vi "HFRR ADV v06.vi"() -> ()   [LabVIEW 2025] (continued)
        n2251 = case shown="\"Acquire\"" w2733 {
          tunnel: w2735 -> [_ w2966]
          frame Default {
            w2965 = 0.0 ("output")
            n2252 = local write "PID-out"(w2965) -> ()
            n2253 = local write "Frequency ( Hz )"(w2965) -> ()
          }
          frame "Acquire" {
            n2254 = stacked-sequence {
              frame #0 {
                n2255 = local read "clk"() -> (w2986:dbl)
                n2256 = local read "Save"() -> (w2982:bool)
                n2257 = Equal?(x=w2986, y=0.0) -> (x = y?=w2983:bool)
                n2258 = case shown="False" "RUN" {
                  tunnel: [w2991 w2999] -> w2969
                  frame False {
                    w2991 = 0.0
                    n2259 = local write "Reinit PID"(TRUE) -> ()
                    n2260 = property on="Stroke" class="DigNum (strict)"("Visible"=TRUE) -> ()  [unwired: 2 in, 2 out]
                    n2261 = property on="Stroke 2" class="DigNum (strict)"("Visible"=FALSE) -> ()  [unwired: 2 in, 2 out]
                    n2262 = local write "String 14"("Test will autostart once parameters reach the set value." ("String 14")) -> ()
                    n2263 = local write "Old Pid Val"(w2991) -> ()
                  }
                  frame True {
                    n2264 = property on="Stroke 2" class="DigNum (strict)"("Visible"=TRUE) -> ()  [unwired: 2 in, 2 out]
                    n2265 = property on="Stroke" class="DigNum (strict)"("Visible"=FALSE) -> ()  [unwired: 2 in, 2 out]
                    n2266 = property on="STOP 2" class="Bool (strict)"("Disabled"=u8 2) -> ()  [unwired: 2 in, 2 out]
                    n2267 = property on="RUN" class="Bool (strict)"("Visible"=TRUE) -> ()  [unwired: 2 in, 2 out]
                    n2268 = local read "PID Ref"() -> (w3010:bool)
                    n2269 = case shown="True" w3010 {
                      tunnel: [w3011 w3027] -> w3009
                      frame False {
                        n2270 = local read "Old Pid Val"() -> (w3011:dbl)
                      }
                      frame True {
                        n2271 = local read "Set Hz"() -> (w3020:dbl)
                        n2272 = local read "Frequency"() -> (w3031:dbl)
                        n2273 = Add(x=w3020, y=10.0) -> (x+y=w3029:dbl)
                        n2274 = Add(x=w3020, y=-10.0 ("Offset")) -> (x+y=w3038:dbl)
                        n2275 = Add(x=w3020, y=-10.0) -> (x+y=w3030:dbl)
                        n2276 = In Range and Coerce(upper limit=w3029, x=w3031, lower limit=w3030) -> (coerced(x)=w3019:dbl)  [unwired: 1 out]
                        n2277 = Or(x="Reinit PID", y="Reinit PID") -> (x .or. y?=w3028:bool)
                        n2278 = Multiply(x=w3038, y=0.1 ("Gain")) -> (x*y=w3017:dbl)
                        n2279 = local read "Elapsed time"() -> (w3024:dbl)
                        n2280 = local read "SPEED OUT:"() -> (w3039:dbl)
                        n2281 = Add(x=w3017, y=1.5) -> (x+y=w3015:dbl)
                        n2282 = call-poly <vilib>:"PID.vi"("reinitialize? (F)"=w3028, "output range"=cluster{"output high":dbl, "output low":dbl} {"output high"=1.0, "output low"=-1.0}, "PID gains"=T10 {"proportional gain (Kc)"=0.0005, "integral time (Ti, min)"=0.001, "derivative time (Td, min)"=0.0} ("Motor PID"), "process variable"=w3019, "setpoint"=w3020) -> ("output"=w3018:dbl)  [unwired: 5 in, 1 out]
                        n2283 = Multiply(x=w3015, y=w3039) -> (x*y=w3014:dbl)
                        n2284 = Greater?(x=w3024, y=0.05) -> (0:w3023:bool)
                        n2285 = case shown="True" w3023 {
                          tunnel: w3018 -> [_ w3041]
                          tunnel: [0.0 ("output") w3041] -> w3021
                          frame False {
                          }
                          frame True {
                            n2286 = local write "Reinit PID"(FALSE ("Reinit PID")) -> ()
                          }
                        }
                        n2287 = Multiply(x=w3014, y=0.8) -> (x*y=w3013:dbl)
                        n2288 = Add(x=w3013, y=w3021) -> (x+y=w3026:dbl)
                        n2289 = flat-sequence {
                          tunnel: [w3044] -> w3027
                          tunnel: w3026 -> [w3044]
                          frame #0 {
                            n2290 = local write "PID Ref"(FALSE ("PID Ref")) -> ()
                          }
                        }
                      }
                    }
                    "Old Pid Val" <- w3009
                    n2291 = local write "String 14"(" Running....." ("String 14")) -> ()
                    n2292 = local read "Set Hz"() -> (w3006:dbl)
                    n2293 = call <vilib>:"Uniform White Noise Waveform.vi"() -> ("signal out"=w3005:waveform(dbl))  [unwired: 10 in, 1 out]
                    n2294 = local read "Freq"() -> (w2998:dbl)
                    n2295 = Add(x=w3006, y=w3005) -> (x+y=w3004:waveform(dbl))
                    n2296 = Multiply(x=w3004, y=ext 0.1) -> (x*y=w3000:waveform(ext))
                    n2297 = Multiply(x=w2998, y=0.9) -> (x*y=w3001:dbl)
                    n2298 = Add(x=w3000, y=w3001) -> (x+y=w2999:waveform(ext))
                  }
                }
                n2299 = And(x=w2983, y=w2982) -> (x .and. y?=w2984:bool)
                n2300 = Not(x="Engage") -> (.not. x?=w2973:bool)
                n2301 = case shown="True" w2984 {
                  frame False {
                  }
                  frame True {
                    n2302 = local write "clk"(10.0 ("clk")) -> ()
                    n2303 = Get Date/Time In Seconds() -> (seconds since 1Jan1904=w3047:timestamp)
                    n2304 = To Double Precision Float(number=w3047) -> (double precision float=w3045:dbl)
                    n2305 = local write "acq timer"(w3045) -> ()
                    n2306 = local write "act save time"(w3045) -> ()
                  }
                }
                n2307 = call "Elapsed Time"("Time Target (s)"="Countdown", "Reset"=w2973) -> ("Elapsed Time (s)"=w2978:dbl, "Time has Elapsed"=w2976:bool)  [unwired: 10 in, 6 out]
                "Countdown 2" <- w2978
                n2308 = Subtract(x=w2978, y=2.0) -> (x-y=w2981:dbl)
                n2309 = Less?(x=w2981, y="Countdown") -> (x < y?=w2979:bool)
                n2310 = And(x=w2979, y=w2976) -> (x .and. y?=w2975:bool)
                n2311 = case shown="True" w2975 {
                  frame False {
                  }
                  frame True {
                    (unwired) dbl[] [] ("History Data")
                    n2312 = local write "Engage"(FALSE ("Engage")) -> ()
                    n2313 = local write "RUN"(TRUE ("RUN")) -> ()
                    n2314 = local read "Humidity ( %RH )"() -> (→"Rh Before":dbl)
                  }
                }
                n2315 = local read "Test \nStatus"() -> (w2971:bool)
                n2316 = Select(t=w2969, s=w2971, f=0.0) -> (s? t:f=w2970:dbl)
                n2317 = local write "Frequency ( Hz )"(w2970) -> ()
                n2318 = local write "Freq"(w2970) -> ()
              }
              frame #1 {
                w3070 = 1000000.0 ("x")
                # "Elapsed time\ncof\nstroke\nAir temp\nTemp\nHumidity"
                # "acq timer\n\nact save time"
                # "convert to microseconds"
                n2319 = local read "COUNT"() -> (w3053:i32)
                n2320 = local read "Rate"() -> (w3066:dbl)
                n2321 = Divide(x=w3070, y=w3066) -> (x/y=w3071:dbl)
                n2322 = Greater Or Equal?(x=w3053, y=250) -> (x >= y?=w3052:bool)
                n2323 = Get Date/Time In Seconds() -> (seconds since 1Jan1904=w3073:timestamp)
                n2324 = case shown="True" w3052 {
                  frame False {
                    n2325 = local read "COUNT"() -> (w3074:i32)
                    n2326 = Increment(x=w3074) -> (x+1=w3075:i32)
                    n2327 = local write "COUNT"(w3075) -> ()
                  }
                  frame True {
                    n2328 = local write "COUNT"(0 ("COUNT")) -> ()
                  }
                }
                n2329 = local read "Samplingtime 2"() -> (w3051:dbl)
                n2330 = local read "act save time"() -> (w3068:dbl)
                n2331 = Divide(x=w3071, y=w3070) -> (x/y=w3069:dbl)
                n2332 = To Double Precision Float(number=w3073) -> (double precision float=w3062:dbl)
                n2333 = Add(x=w3068, y=w3051) -> (x+y=w3067:dbl)
                n2334 = local read "acq timer"() -> (w3072:dbl)
                n2335 = local read "COUNT"() -> (w3055:i32)
                n2336 = Greater Or Equal?(x=w3062, y=w3067) -> (x >= y?=w3050:bool)
                n2337 = Multiply(x=w3069, y=w3055) -> (x*y=w3061:dbl)
                n2338 = Subtract(x=w3062, y=w3072) -> (x-y=w3064:dbl)
                n2339 = local read "Save"() -> (w3065:bool)
                n2340 = Add(x=w3064, y=w3061) -> (x+y=w3048:dbl)
                "Elapsed time 3" <- w3048
                n2341 = And(x=w3050, y=w3065) -> (x .and. y?=w3063:bool)
                n2342 = Divide(x=w3048, y=60.0) -> (x/y=w3059:dbl)
                n2343 = local read "Test \nStatus"() -> (w3049:bool)
                n2344 = local read "clk"() -> (w3056:dbl)
                n2345 = case shown="True" w3063 {
                  tunnel: w3062 -> [_ w3164]
                  tunnel: [FALSE ("Boolean 2") TRUE ("Boolean 2")] -> _
                  frame False {
                  }
                  frame True {
                    w3111 = ";" ("Substring")
                    # "Pid out/\nFreq response value"
                    n2346 = local read "FILE"() -> (w3105:string)
                    n2347 = call "file check.vi"("file name in"=w3105) -> ("error out"=w3108:errorcluster, "file name out"=w3103:string)  [unwired: 9 in]
                    n2348 = call "FILE PATH CREATION.vi"("error in"=w3108, "FILE NAME :"=w3103) -> ("FILE OUT"=w3106:path)  [unwired: 8 in, 1 out]
                    n2349 = Concatenate Strings(w3103, ".dgf" ("Substring")) -> (w3107:string)
                    n2350 = local write "act save time"(w3164) -> ()
                    n2351 = local read "Set Strk"() -> (w3135:dbl)
                    n2352 = local read "Stroke"() -> (w3126:dbl)
                    n2353 = local read "FF 2"() -> (w3122:dbl)
                    "Frictional Force ( N )" <- w3122
                    "Frictional Force ( N )" <- w3122
                    n2354 = Build Path(base path=w3106, name or relative path=w3107) -> (appended path=w3102:path)
                    n2355 = local write "FF 3"(w3122) -> ()
                    n2356 = Subtract(x=w3126, y=w3135) -> (x-y=w3132:dbl)
                    n2357 = local read "COF 2"() -> (w3117:dbl)
                    "cof" <- w3117
                    "Coefficient of Friction" <- w3117
                    "COF 4" <- w3117
                    "Coefficient of Friction" <- w3117
                    n2358 = local write "COF 3"(w3117) -> ()
                    n2359 = Multiply(x=w3132, y=0.05) -> (x*y=w3134:dbl)
                    n2360 = local read "TEMP"() -> (w3121:dbl)
                    "Temp" <- w3121
                    "Temperature ( Deg C )" <- w3121
                    n2361 = Add(x=w3134, y=w3135) -> (x+y=w3115:dbl)
                    "Stroke Ln" <- w3115
                    "Disp" <- w3115
                    n2362 = local read "ecr"() -> (w3118:dbl)
                    "ecr 2" <- w3118
                    "Electrical Contact Resistance ( % )" <- w3118
                    "ecr 4" <- w3118
                    n2363 = local read "Humidity ( %RH )"() -> (w3120:dbl)
                    "Humidity ( %RH )" <- w3120
                    "Humidity ( %RH )" <- w3120
                    n2364 = local read "Frequency ( Hz )"() -> (w3128:dbl)
                    n2365 = local read "Elapsed time"() -> (w3157:dbl)
                    n2366 = local read "AIR TEMP"() -> (w3125:dbl)
                    n2367 = local write "ecr 3"(w3118) -> ()
                    n2368 = local read "PID-out"() -> (w3131:dbl)
                    n2369 = local write "Temperature ( Deg C )"(w3121) -> ()
                    n2370 = local write "Electrical Contact Resistance ( % )"(w3118) -> ()
                    n2371 = Number To Fractional String(number=w3115, width (-)=i16 9 ("precision (6)"), precision (6)=i16 6) -> (F-format string=w3150:string)  [unwired: 1 in]
                    n2372 = Number To Fractional String(number=w3125, width (-)=i16 9 ("precision (6)"), precision (6)=i16 3) -> (F-format string=w3149:string)  [unwired: 1 in]
                    n2373 = Number To Fractional String(number=w3121, width (-)=i16 9 ("precision (6)"), precision (6)=i16 3) -> (F-format string=w3146:string)  [unwired: 1 in]
                    n2374 = Number To Fractional String(number=w3120, width (-)=i16 9 ("precision (6)"), precision (6)=i16 3) -> (F-format string=w3143:string)  [unwired: 1 in]
                    n2375 = Number To Fractional String(number=w3118, width (-)=i16 9 ("precision (6)"), precision (6)=i16 3) -> (F-format string=w3140:string)  [unwired: 1 in]
                    n2376 = Number To Fractional String(number=w3131, width (-)=i16 9 ("precision (6)"), precision (6)=i16 3) -> (F-format string=w3136:string)  [unwired: 1 in]
                    n2377 = Number To Fractional String(number=w3128, width (-)=i16 9 ("precision (6)"), precision (6)=i16 3) -> (F-format string=w3127:string)  [unwired: 1 in]
                    n2378 = Number To Fractional String(number=w3117, width (-)=i16 9 ("precision (6)"), precision (6)=i16 6) -> (F-format string=w3158:string)  [unwired: 1 in]
                    n2379 = Number To Fractional String(number=w3157, width (-)=i16 14 ("precision (6)"), precision (6)=i16 3) -> (F-format string=w3159:string)  [unwired: 1 in]
                    n2380 = Bundle("y"=1.02, w3115, "y"=0.98) -> (w3119:cluster{"y":dbl, dbl, "y":dbl})  [unwired: 1 in]
                    n2381 = Number To Fractional String(number="Ambient Humidity :", width (-)=i16 9 ("precision (6)"), precision (6)=i16 6) -> (F-format string=w3109:string)  [unwired: 1 in]
                    n2382 = local read "RUN"() -> (w3116:bool)
                    n2383 = case shown="True" w3116 {
                      tunnel: w3119 -> [_ w3169]
                      tunnel: w3115 -> [_ w3168]
                      tunnel: w3115 -> [_ w3167]
                      tunnel: w3115 -> [_ w3166]
                      frame False {
                      }
                      frame True {
                        "Stroke ( mm )" <- w3169
                        "Stroke ( mm )" <- w3169
                        "Stroke 4" <- w3168
                        "Stroke 3" <- w3167
                        "Stroke 2" <- w3166
                      }
                    }
                    n2384 = Concatenate Strings(w3159, w3111, w3158, w3111, w3150, w3111, w3149, w3111, w3146, w3111, w3143, w3111, w3140, w3111, w3136, w3111, w3127, w3111, w3109, "\r") -> (w3156:string)
                    n2385 = call <vilib>:"Write Characters To File.vi"("append to file? (new file:F)"=TRUE, "character string"=w3156, "file path (dialog if empty)"=w3102) -> ()  [unwired: 2 in, 1 out]
                    "refresh flag" <- TRUE ("refresh flag")
                  }
                }
                n2386 = Equal?(x=w3056, y=10.0) -> (x = y?=w3058:bool)
                n2387 = case shown="True" w3049 {
                  tunnel: w3059 -> [_ w3082]
                  tunnel: w3064 -> [_ w3093]
                  tunnel: [0.0 w3089] -> _
                  tunnel: w3058 -> [_ w3088]
                  tunnel: [0.0 w3087] -> _
                  tunnel: w3048 -> [_ w3087]
                  tunnel: w3062 -> [w3078 _]
                  frame False {
                    n2388 = local write "acq timer"(w3078) -> ()
                    n2389 = local write "Test Duration Status"(0.0 ("Test Duration Status")) -> ()
                  }
                  frame True {
                    n2390 = local read "Set Hz"() -> (w3090:dbl)
                    n2391 = local write "Elapsed time"(w3082) -> ()
                    n2392 = local read "test time"() -> (w3081:dbl)
                    n2393 = Multiply(x=w3093, y=w3090) -> (x*y=w3092:dbl)
                    n2394 = case shown="False" w3088 {
                      tunnel: w3092 -> [w3094 _]
                      tunnel: [w3094 1.0] -> w3089
                      frame False {
                        n2395 = local write "Cycles elapsed"(w3094) -> ()
                      }
                      frame True {
                      }
                    }
                    n2396 = Greater?(x=w3082, y=w3081) -> (0:w3091:bool)
                    n2397 = Subtract(x=w3081, y=w3082) -> (x-y=w3086:dbl)
                    "time" <- w3086
                    n2398 = case shown="True" w3091 {
                      frame False {
                      }
                      frame True {
                        n2399 = local write "RUN"(FALSE ("OK Button 2")) -> ()
                        n2400 = property on="STOP 2" class="Bool (strict)"("Disabled"=u8 0) -> ()  [unwired: 2 in, 2 out]
                        n2401 = local read "Humidity ( %RH )"() -> (→"Rh After":dbl)
                        n2402 = local write "Heater Button"(FALSE ("Heater Button")) -> ()
                        n2403 = local write "Humidity"(FALSE ("Humidity")) -> ()
                      }
                    }
                    n2404 = local write "Time Remaining"(w3086) -> ()
                    n2405 = Divide(x=w3082, y=w3081) -> (x/y=w3085:dbl)
                    n2406 = Multiply(x=w3085, y=100.0) -> (x*y=w3083:dbl)
                    n2407 = local write "Test Duration Status"(w3083) -> ()
                  }
                }
              }
              frame #2 {
                n2408 = case shown="True" "Heater Button" {
                  tunnel: [0.0 ("output") w3191] -> w3170
                  frame False {
                    w3172 = TRUE ("tmpchk")
                    n2409 = local read "TEMP"() -> (w3173:dbl)
                    n2410 = local write "Temp ini"(w3173) -> ()
                    n2411 = local write "Reset 4"(w3172) -> ()
                    n2412 = local write "tmpchk"(w3172) -> ()
                    n2413 = local write "reinit"(TRUE ("reinit")) -> ()
                  }
                  frame True {
                    # "Logic to turn off\nthe heater when \ntemp is not rising.\nTime - 60 sec\nDelta t- 5°c"
                    n2414 = local read "Temp ini"() -> (w3179:dbl)
                    n2415 = Less?(x=w3179, y=53.0) -> (x < y?=w3177:bool)
                    n2416 = And(x="tmpchk", y=w3177) -> (x .and. y?=w3180:bool)
                    n2417 = case shown="True" w3180 {
                      frame False {
                      }
                      frame True {
                        n2418 = call "Elapsed Time8"("Time Target (s)"=300.0, "Reset"="Reset 4") -> ("Time has Elapsed"=w3196:bool)  [unwired: 10 in, 7 out]
                        n2419 = flat-sequence {
                          tunnel: w3196 -> [_]
                          frame #0 {
                            n2420 = local write "Reset 4"(FALSE ("Reset 4")) -> ()
                          }
                        }
                        n2421 = case shown="True" w3196 {
                          frame False {
                          }
                          frame True {
                            n2422 = local read "Temp ini"() -> (w3203:dbl)
                            n2423 = Add(x=w3203, y=5.0) -> (x+y=w3201:dbl)
                            n2424 = local read "TEMP"() -> (w3204:dbl)
                            n2425 = Greater?(x=w3204, y=w3201) -> (0:w3202:bool)
                            n2426 = case shown="False" w3202 {
                              frame False {
                                n2427 = local write "Heater Button"(FALSE ("Heater Button")) -> ()
                              }
                              frame True {
                                n2428 = local write "tmpchk"(FALSE ("tmpchk")) -> ()
                              }
                            }
                          }
                        }
                      }
                    }
                    n2429 = local read "Set Temp"() -> (w3188:dbl)
                    n2430 = local read "TEMP"() -> (w3182:dbl)
                    n2431 = call-poly <vilib>:"PID.vi"("reinitialize? (F)"="reinit", "output range"="output range", "dt (s)"=-1.0, "PID gains"="Temp PID gains", "process variable"=w3182, "setpoint"=w3188) -> ("output"=w3185:dbl)  [unwired: 4 in, 1 out]
                    n2432 = Subtract(x=w3188, y=w3182) -> (x-y=w3190:dbl)
                    n2433 = Add(x=w3188, y=0.5) -> (x+y=w3186:dbl)
                    n2434 = Greater Or Equal?(x=w3182, y=w3186) -> ()  [unwired: 1 out]
                    n2435 = Select(t=0.0, s=FALSE, f=w3185) -> (s? t:f=w3184:dbl)
                    "PID output" <- w3184
                    n2436 = flat-sequence {
                      tunnel: w3184 -> [w3207]
                      tunnel: [w3207] -> w3191
                      frame #0 {
                        n2437 = local write "reinit"(FALSE ("reinit")) -> ()
                      }
                    }
                    n2438 = Bundle(w3190, "output"=w3184, "TEMP"=w3182) -> (→"gTEMP 3":cluster{dbl, "output":dbl, "TEMP":dbl})  [unwired: 1 in]
                  }
                }
                "PID-out" <- w3170
              }
              frame #3 {
                n2439 = local read "TEMP"() -> (w3209:dbl)
                n2440 = Greater Or Equal?(x=w3209, y="Set Temp 2") -> (x >= y?=w3214:bool)
                n2441 = case shown="True" w3214 {
                  tunnel: [FALSE TRUE] -> w3212
                  frame False {
                  }
                  frame True {
                  }
                }
                "Status 13" <- w3212
                n2442 = And(x=w3212, y="trip1 8") -> (x .and. y?=w3211:bool)
                n2443 = case shown="True" w3211 {
                  frame False {
                  }
                  frame True {
                    w3215 = FALSE ("OK Button 2")
                    n2444 = local write "RUN"(w3215) -> ()
                    n2445 = local write "Heater Button"(w3215) -> ()
                  }
                }
              }
            }
            n2446 = case shown="False" w2966 {
              frame False {
                n2447 = disable-structure shown="Enabled" {
                  frame Enabled {
                    n2448 = stacked-sequence {
                      frame #0 {
                        n2449 = local write "RUN"(FALSE ("OK Button 2")) -> ()
                      }
                      frame #1 {
                      }
                    }
                  }
                  frame Disabled {
                  }
                }
              }
              frame True {
              }
            }
          }
        }
        n2450 = local read "airtempflg"() -> (w2758:bool)
        n2451 = Or(x=w2758, y=w2756) -> (x .or. y?=w2759:bool)
        n2452 = Insert Into Array(array=string[] ["Air Temperature has reached set value,", "Humidity has reached set value,", "Sample Temperaturehas reached set value,", ""], index=0, new element="") -> (w2744:string[])
        n2453 = disable-structure shown="Disabled" {
          disable-tunnel: w2759 -> [w2836 _]
          disable-tunnel: w2754 -> [w2835 _]
          disable-tunnel: w2752 -> [w2834 _]
          frame Disabled {
            n2454 = Compound Arithmetic op=AND(w2836, w2835, w2834) -> ()  [unwired: 1 out]
            n2455 = case shown="True" {
              selector: _ -> [_ _]
              frame False {
              }
              frame True {
                w2837 = FALSE ("autostrtflg")
                n2456 = local write "RUN"(TRUE ("RUN")) -> ()
                n2457 = local write "autostrtflg"(w2837) -> ()
                n2458 = local write "autostart"(w2837) -> ()
                n2459 = local write "String 14"(" Running....." ("String 14")) -> ()
              }
            }
          }
          frame Enabled {
          }
        }
        n2460 = Build Array(w2749, w2748, w2747) -> (w2745:i32[])
        n2461 = for {
          tunnel: w2745 -> [w2887] mode=indexing
          tunnel: w2744 -> [w2886]
          shift-right: [w2883] -> w2743
          shift-left: "" -> [w2885]
          n2462 = Index Array(array=w2886, index=w2887) -> (element=w2884:string)
          n2463 = Concatenate Strings(w2884, w2885) -> (w2883:string)
        }
        n2464 = local write "autostart 2"(w2743) -> ()
        n2465 = local read "Reset Graph"() -> (w2732:bool)
        n2466 = case shown="True" w2732 {
          selector: w2732 -> [_ w2786]
          frame False {
          }
          frame True {
            w2800 = 0.0 ("X Scale.Range:Maximum")
            n2467 = Not(x=w2786) -> (.not. x?=w2785:bool)
            n2468 = local write "Reset Graph"(w2785) -> ()
            n2469 = property on="Electrical Contact Resistance ( % )" class="WFChart (strict)"("XScale.Maximum"=600.0 ("X Scale.Range:Maximum"), "XScale.Minimum"=0.0 ("X Scale.Range:Minimum"), "YScale.Maximum"=100.0 ("Y Scale.Range:Maximum"), "YScale.Minimum"=0.0 ("Y Scale.Range:Minimum")) -> ()  [unwired: 2 in, 2 out]
            n2470 = property on="Frictional Force ( N )" class="WFChart (strict)"("XScale.Maximum"=600.0 ("X Scale.Range:Maximum"), "XScale.Minimum"=0.0 ("X Scale.Range:Minimum"), "YScale.Maximum"=100.0 ("Y Scale.Range:Maximum"), "YScale.Minimum"=0.0 ("Y Scale.Range:Minimum")) -> ()  [unwired: 2 in, 2 out]
            n2471 = property on="Temperature ( Deg C )" class="WFChart (strict)"("XScale.Maximum"=600.0 ("X Scale.Range:Maximum"), "XScale.Minimum"=0.0 ("X Scale.Range:Minimum"), "YScale.Maximum"=100.0 ("Y Scale.Range:Maximum"), "YScale.Minimum"=0.0 ("Y Scale.Range:Minimum")) -> ()  [unwired: 2 in, 2 out]
            n2472 = property on="Humidity ( %RH )" class="WFChart (strict)"("XScale.Maximum"=600.0 ("X Scale.Range:Maximum"), "XScale.Minimum"=0.0 ("X Scale.Range:Minimum"), "YScale.Maximum"=100.0 ("Y Scale.Range:Maximum"), "YScale.Minimum"=0.0 ("Y Scale.Range:Minimum")) -> ()  [unwired: 2 in, 2 out]
            n2473 = property on="Stroke ( mm )" class="WFChart (strict)"("XScale.Maximum"=600.0 ("X Scale.Range:Maximum"), "XScale.Minimum"=0.0 ("X Scale.Range:Minimum"), "YScale.Maximum"=100.0 ("Y Scale.Range:Maximum"), "YScale.Minimum"=0.0 ("Y Scale.Range:Minimum")) -> ()  [unwired: 2 in, 2 out]
            n2474 = property on="Coefficient of Friction" class="WFChart (strict)"("XScale.Maximum"=600.0 ("X Scale.Range:Maximum"), "XScale.Minimum"=0.0 ("X Scale.Range:Minimum"), "YScale.Maximum"=100.0 ("Y Scale.Range:Maximum"), "YScale.Minimum"=0.0 ("Y Scale.Range:Minimum")) -> ()  [unwired: 2 in, 2 out]
            n2475 = property on="Electrical Contact Resistance ( % )" class="WFChart (strict)"("XScale.Minimum"=0.0 ("X Scale.Range:Minimum"), "XScale.Maximum"=600.0 ("X Scale.Range:Maximum"), "YScale.Minimum"=0.0 ("Y Scale.Range:Minimum"), "YScale.Maximum"=100.0 ("Y Scale.Range:Maximum")) -> ()  [unwired: 2 in, 2 out]
            n2476 = property on="Temperature ( Deg C )" class="WFChart (strict)"("XScale.Minimum"=0.0 ("X Scale.Range:Minimum"), "XScale.Maximum"=600.0 ("X Scale.Range:Maximum"), "YScale.Minimum"=0.0 ("Y Scale.Range:Minimum"), "YScale.Maximum"=100.0 ("Y Scale.Range:Maximum")) -> ()  [unwired: 2 in, 2 out]
            n2477 = property on="Coefficient of Friction" class="WFChart (strict)"("XScale.Minimum"=0.0 ("X Scale.Range:Minimum"), "XScale.Maximum"=600.0 ("X Scale.Range:Maximum"), "YScale.Maximum"=1.0 ("X Scale.Range:Minimum"), "YScale.Minimum"=0.0 ("X Scale.Range:Minimum")) -> ()  [unwired: 2 in, 2 out]
            n2478 = property on="Frictional Force ( N )" class="WFChart (strict)"("XScale.Maximum"=600.0 ("X Scale.Range:Maximum"), "XScale.Minimum"=w2800, "YScale.Maximum"=10.0 ("Y Scale.Range:Maximum"), "YScale.Minimum"=w2800) -> ()  [unwired: 2 in, 2 out]
            n2479 = property on="Stroke ( mm )" class="WFChart (strict)"("XScale.Maximum"=600.0 ("X Scale.Range:Maximum"), "XScale.Minimum"=0.0 ("X Scale.Range:Minimum"), "YScale.Maximum"=100.0 ("Y Scale.Range:Maximum"), "YScale.Minimum"=0.0 ("Y Scale.Range:Minimum")) -> ()  [unwired: 2 in, 2 out]
            n2480 = property on="Humidity ( %RH )" class="WFChart (strict)"("XScale.Maximum"=600.0 ("X Scale.Range:Maximum"), "XScale.Minimum"=0.0 ("X Scale.Range:Minimum"), "YScale.Maximum"=100.0 ("Y Scale.Range:Maximum"), "YScale.Minimum"=0.0 ("Y Scale.Range:Minimum")) -> ()  [unwired: 2 in, 2 out]
          }
        }
      }
      frame "Compare Files" {
        # "Elapsed time\ncof\nstroke\nAir temp\nTemp\nHumidity"
        n2481 = case shown="True" "RSTV1 2" {
          frame False {
          }
          frame True {
            n2482 = property on="Humidity ( %Rh )" class="XYGraph (strict)"("Y Scale.Display Format:Precision"=u8 0 ("Y Scale.Format & Precision:Precision")) -> ()  [unwired: 2 in, 2 out]
            n2483 = property on="Humidity ( %Rh )" class="XYGraph (strict)"("X Scale.Range:Minimum"=0.0, "X Scale.Range:Maximum"=75.0, "Y Scale.Range:Minimum"=48.0, "Y Scale.Range:Maximum"=58.0) -> ()  [unwired: 2 in, 2 out]
          }
        }
        n2484 = case shown="True" "RST CP 2" {
          frame False {
          }
          frame True {
            n2485 = property on="XY Graph 13" class="XYGraph (strict)"("Y Scale.Display Format:Precision"=u8 0 ("Y Scale.Format & Precision:Precision")) -> ()  [unwired: 2 in, 2 out]
            n2486 = property on="XY Graph 13" class="XYGraph (strict)"("X Scale.Range:Minimum"=0.0, "X Scale.Range:Maximum"=75.0, "Y Scale.Range:Minimum"=0.0, "Y Scale.Range:Maximum"=100.0) -> ()  [unwired: 2 in, 2 out]
          }
        }
        n2487 = case shown="True" "RST CP" {
          frame False {
          }
          frame True {
            n2488 = property on="Sample Temperature ( °C )" class="XYGraph (strict)"("Y Scale.Display Format:Precision"=u8 2 ("Y Scale.Format & Precision:Precision")) -> ()  [unwired: 2 in, 2 out]
            n2489 = property on="Sample Temperature ( °C )" class="XYGraph (strict)"("X Scale.Range:Minimum"=0.0, "X Scale.Range:Maximum"=75.0, "Y Scale.Range:Minimum"=58.0, "Y Scale.Range:Maximum"=62.0) -> ()  [unwired: 2 in, 2 out]
          }
        }
        n2490 = case shown="True" "RSTV1 3" {
          frame False {
          }
          frame True {
            n2491 = property on="Air Temperature  ( °C )" class="XYGraph (strict)"("Y Scale.Display Format:Precision"=u8 2 ("Y Scale.Format & Precision:Precision")) -> ()  [unwired: 2 in, 2 out]
            n2492 = property on="Air Temperature  ( °C )" class="XYGraph (strict)"("X Scale.Range:Minimum"=0.0 ("Y Scale.Range:Minimum"), "X Scale.Range:Maximum"=75.0 ("Y Scale.Range:Maximum"), "Y Scale.Range:Minimum"=20.0 ("X Scale.Range:Minimum"), "Y Scale.Range:Maximum"=26.0 ("X Scale.Range:Maximum")) -> ()  [unwired: 2 in, 2 out]
          }
        }
        n2493 = case shown="True" "RSTV1 4" {
          frame False {
          }
          frame True {
            n2494 = property on="Stroke ( mm )" class="XYGraph (strict)"("Y Scale.Display Format:Precision"=u8 2 ("Y Scale.Format & Precision:Precision")) -> ()  [unwired: 2 in, 2 out]
            n2495 = property on="Stroke ( mm )" class="XYGraph (strict)"("X Scale.Range:Minimum"=0.0 ("Y Scale.Range:Maximum"), "X Scale.Range:Maximum"=75.0 ("X Scale.Range:Minimum"), "Y Scale.Range:Minimum"=0.98, "Y Scale.Range:Maximum"=1.02) -> ()  [unwired: 2 in, 2 out]
          }
        }
        n2496 = case shown="True" "rstv2" {
          frame False {
          }
          frame True {
            n2497 = property on="Coefficient Of Friction" class="XYGraph (strict)"("Y Scale.Display Format:Precision"=u8 3 ("Y Scale.Format & Precision:Precision")) -> ()  [unwired: 2 in, 2 out]
            n2498 = property on="Coefficient Of Friction" class="XYGraph (strict)"("X Scale.Range:Minimum"=0.0 ("Y Scale.Range:Maximum"), "X Scale.Range:Maximum"=75.0, "Y Scale.Range:Minimum"=0.0, "Y Scale.Range:Maximum"=1.0 ("X Scale.Range:Minimum")) -> ()  [unwired: 2 in, 2 out]
          }
        }
        n2499 = case shown="True" "RST CP 3" {
          frame False {
          }
          frame True {
            n2500 = property on="Air Temp ( °C ) vs Humidity ( % Rh )" class="XYGraph (strict)"("X Scale.Range:Minimum"=18.0, "X Scale.Range:Maximum"=28.0 ("X Scale.Range:Minimum"), "Y Scale.Range:Minimum"=30.0 ("X Scale.Range:Minimum"), "Y Scale.Range:Maximum"=70.0 ("X Scale.Range:Minimum")) -> ()  [unwired: 2 in, 2 out]
          }
        }
        n2501 = case shown="True" "OPEN 1" {
          frame False {
          }
          frame True {
            (unwired) 0  # existing file
            w3479 = "Choose a datalog file to open"  # prompt
            n2502 = local write "OPEN 1"(FALSE ("OPEN 1")) -> ()
            n2503 = String To Path(string="C:\\LAB-IQ\\Data\\") -> (path=w3464:path)
            n2504 = File Dialog(6:"*.dgf" ("pattern"), 7:w3479, 11:w3464) -> (0:w3462:errorcluster, 3:w3470:path)  [unwired: 4 in, 2 out]
            n2505 = Unbundle(w3462) -> ()  [unwired: 3 out]
            n2506 = Strip Path(path=w3470) -> (name=w3469:string)  [unwired: 1 out]
            n2507 = Path To String(path=w3470) -> (string=w3465:string)
            "string1" <- w3465
            n2508 = Match Pattern(string=w3469, regular expression=".dgf") -> (before substring=→"String Control":string)  [unwired: 1 in, 3 out]
            n2509 = Match Pattern(string=w3465, regular expression=".dgf" ("substring (\"\")")) -> (before substring=w3475:string)  [unwired: 1 in, 3 out]
            n2510 = Concatenate Strings(w3475, ".duf" ("Substring")) -> (w3471:string)
            n2511 = String To Path(string=w3471) -> (path=w3476:path)
            n2512 = call <vilib>:"Read Characters From File.vi"("file path (dialog if empty)"=w3476, "start of read offset (chars.:0)"=60 ("start of read offset (chars.: 0)")) -> ("character string"=→"String Control 2":string)  [unwired: 4 in, 3 out]
          }
        }
        n2513 = case shown="True" "OPEN 2" {
          frame False {
          }
          frame True {
            (unwired) 0  # existing file
            w3497 = "Choose a datalog file to open"  # prompt
            n2514 = local write "OPEN 2"(FALSE ("OPEN 1")) -> ()
            n2515 = String To Path(string="C:\\LAB-IQ\\Data\\") -> (path=w3482:path)
            n2516 = File Dialog(6:"*.dgf" ("pattern"), 7:w3497, 11:w3482) -> (0:w3480:errorcluster, 3:w3488:path)  [unwired: 4 in, 2 out]
            n2517 = Unbundle(w3480) -> ()  [unwired: 3 out]
            n2518 = Strip Path(path=w3488) -> (name=w3486:string)  [unwired: 1 out]
            n2519 = Path To String(path=w3488) -> (string=w3483:string)
            "string1 2" <- w3483
            n2520 = Match Pattern(string=w3486, regular expression=".dgf") -> (before substring=→"String Control 3":string)  [unwired: 1 in, 3 out]
            n2521 = Match Pattern(string=w3483, regular expression=".dgf" ("substring (\"\")")) -> (before substring=w3494:string)  [unwired: 1 in, 3 out]
            n2522 = Concatenate Strings(w3494, ".duf" ("Substring")) -> (w3491:string)
            n2523 = String To Path(string=w3491) -> (path=w3489:path)
            n2524 = call <vilib>:"Read Characters From File.vi"("file path (dialog if empty)"=w3489, "start of read offset (chars.:0)"=60 ("start of read offset (chars.: 0)")) -> ("character string"=→"String Control 4":string)  [unwired: 4 in, 3 out]
          }
        }
        n2525 = case shown="True" "OPEN 3" {
          frame False {
          }
          frame True {
            (unwired) 0  # existing file
            w3515 = "Choose a datalog file to open"  # prompt
            n2526 = local write "OPEN 3"(FALSE ("OPEN 1")) -> ()
            n2527 = String To Path(string="C:\\LAB-IQ\\Data\\") -> (path=w3500:path)
            n2528 = File Dialog(6:"*.dgf" ("pattern"), 7:w3515, 11:w3500) -> (0:w3498:errorcluster, 3:w3506:path)  [unwired: 4 in, 2 out]
            n2529 = Unbundle(w3498) -> ()  [unwired: 3 out]
            n2530 = Strip Path(path=w3506) -> (name=w3504:string)  [unwired: 1 out]
            n2531 = Path To String(path=w3506) -> (string=w3501:string)
            "string1 3" <- w3501
            n2532 = Match Pattern(string=w3504, regular expression=".dgf") -> (before substring=→"String Control 5":string)  [unwired: 1 in, 3 out]
            n2533 = Match Pattern(string=w3501, regular expression=".dgf" ("substring (\"\")")) -> (before substring=w3511:string)  [unwired: 1 in, 3 out]
            n2534 = Concatenate Strings(w3511, ".duf" ("Substring")) -> (w3508:string)
            n2535 = String To Path(string=w3508) -> (path=w3512:path)
            n2536 = call <vilib>:"Read Characters From File.vi"("file path (dialog if empty)"=w3512, "start of read offset (chars.:0)"=60 ("start of read offset (chars.: 0)")) -> ("character string"=→"String Control 6":string)  [unwired: 4 in, 3 out]
          }
        }
        n2537 = case shown="True" "OPEN 4" {
          frame False {
          }
          frame True {
            (unwired) 0  # existing file
            w3533 = "Choose a datalog file to open"  # prompt
            n2538 = local write "OPEN 4"(FALSE ("OPEN 1")) -> ()
            n2539 = String To Path(string="C:\\LAB-IQ\\Data\\") -> (path=w3518:path)
            n2540 = File Dialog(6:"*.dgf" ("pattern"), 7:w3533, 11:w3518) -> (0:w3516:errorcluster, 3:w3524:path)  [unwired: 4 in, 2 out]
            n2541 = Unbundle(w3516) -> ()  [unwired: 3 out]
            n2542 = Strip Path(path=w3524) -> (name=w3522:string)  [unwired: 1 out]
            n2543 = Path To String(path=w3524) -> (string=w3519:string)
            "string1 4" <- w3519
            n2544 = Match Pattern(string=w3522, regular expression=".dgf") -> (before substring=→"String Control 7":string)  [unwired: 1 in, 3 out]
            n2545 = Match Pattern(string=w3519, regular expression=".dgf" ("substring (\"\")")) -> (before substring=w3529:string)  [unwired: 1 in, 3 out]
            n2546 = Concatenate Strings(w3529, ".duf" ("Substring")) -> (w3526:string)
            n2547 = String To Path(string=w3526) -> (path=w3530:path)
            n2548 = call <vilib>:"Read Characters From File.vi"("file path (dialog if empty)"=w3530, "start of read offset (chars.:0)"=60 ("start of read offset (chars.: 0)")) -> ("character string"=→"String Control 8":string)  [unwired: 4 in, 3 out]
          }
        }
      }
      frame "About" {
        # "Elapsed time\ncof\nstroke\nmean pos\nTemp\nHumidity"
        n2549 = disable-structure shown="Disabled" {
          frame Disabled {
            n2550 = case shown="True" "Export" {
              frame False {
              }
              frame True {
                w3555 = "                                      " ("string")
                w3557 = "\r"
                (unwired) i16 6 ("width (-)")
                w3634 = "\r"
                w3566 = "\r"
                n2551 = local write "Export"(FALSE ("Export")) -> ()
                n2552 = local read "String 29"() -> (w3603:string)
                n2553 = local read "String 34"() -> (w3591:string)
                n2554 = local read "String 35"() -> (w3586:string)
                n2555 = local read "String 37"() -> (w3582:string)
                n2556 = local read "String 36"() -> (w3579:string)
                n2557 = local read "String 38"() -> (w3576:string)
                n2558 = local read "String 39"() -> (w3573:string)
                n2559 = Match Pattern(string=w3603, regular expression=".dwm") -> (before substring=w3599:string)  [unwired: 1 in, 3 out]
                "before substring" <- w3599
                n2560 = local read "S 38"() -> (w3594:string)
                n2561 = local read "S 39"() -> (w3587:string)
                n2562 = local read "Temperature before test 2"() -> (w3623:dbl)
                n2563 = local read "Temperature after test 2"() -> (w3628:dbl)
                n2564 = local read "Humidity before test 2"() -> (w3609:dbl)
                n2565 = local read "Humidity after test 2"() -> (w3624:dbl)
                n2566 = local read "MWSD 2"() -> (w3620:dbl)
                n2567 = local read "WS1.4 2"() -> (w3636:dbl)
                n2568 = local read "HCF 2"() -> (w3632:dbl)
                n2569 = local read "AVP 2"() -> (w3621:dbl)
                n2570 = Concatenate Strings("1," ("string"), w3594) -> (w3593:string)
                n2571 = Concatenate Strings("2," ("string"), w3591) -> (w3590:string)
                n2572 = Concatenate Strings("3," ("string"), w3587) -> (w3589:string)
                n2573 = Concatenate Strings("4," ("string"), w3586) -> (w3585:string)
                n2574 = Concatenate Strings("5," ("string"), w3582) -> (w3583:string)
                n2575 = Concatenate Strings("6," ("string"), w3579) -> (w3580:string)
                n2576 = Concatenate Strings("7," ("string"), w3576) -> (w3577:string)
                n2577 = Concatenate Strings("8," ("string"), w3573) -> (w3574:string)
                n2578 = local read "Sample ID"() -> (w3641:string)
                n2579 = case shown="\"xlx\"" "Select File Type" {
                  tunnel: w3599 -> [w3644 w3646 w3648]
                  tunnel: [w3642 w3647 w3649] -> w3598
                  frame "xlx" {
                    n2580 = Concatenate Strings(w3644, ".xls" ("string")) -> (w3642:string)
                  }
                  frame "csv" {
                    n2581 = Concatenate Strings(w3646, ".csv" ("string")) -> (w3647:string)
                  }
                  frame "txt" {
                    n2582 = Concatenate Strings(w3648, ".txt" ("string")) -> (w3649:string)
                  }
                }
                n2583 = local read "Test Date"() -> (w3640:string)
                n2584 = local read "String 45"() -> (w3554:string)
                n2585 = local read "String 31"() -> (w3639:string)
                n2586 = local read "String 32"() -> (w3638:string)
                n2587 = local read "TITTLE"() -> (w3562:string)
                n2588 = Number To Fractional String(number=w3609, width (-)=i16 6, precision (6)=i16 2) -> (F-format string=w3608:string)  [unwired: 1 in]
                n2589 = Number To Fractional String(number=w3623, width (-)=i16 6, precision (6)=i16 2) -> (F-format string=w3629:string)  [unwired: 1 in]
                n2590 = Number To Fractional String(number=w3624, width (-)=i16 6, precision (6)=i16 2) -> (F-format string=w3622:string)  [unwired: 1 in]
                n2591 = Number To Fractional String(number=w3628, width (-)=i16 6, precision (6)=i16 2) -> (F-format string=w3627:string)  [unwired: 1 in]
                n2592 = Number To Fractional String(number=w3620, width (-)=i16 6, precision (6)=i16 2) -> (F-format string=w3618:string)  [unwired: 1 in]
                n2593 = Number To Fractional String(number=w3621, width (-)=i16 6, precision (6)=i16 2) -> (F-format string=w3619:string)  [unwired: 1 in]
                n2594 = Number To Fractional String(number=w3632, width (-)=i16 6, precision (6)=i16 2) -> (F-format string=w3633:string)  [unwired: 1 in]
                n2595 = Number To Fractional String(number=w3636, precision (6)=i16 2) -> (F-format string=w3637:string)  [unwired: 2 in]
                n2596 = local read "s.NO"() -> (w3556:string)
                n2597 = Concatenate Strings("=" ("string"), w3562) -> (w3561:string)
                n2598 = Concatenate Strings("S.No," ("string"), "                                       Parameters" ("string")) -> (w3567:string)
                n2599 = Concatenate Strings(w3634, w3593, w3608, w3634, w3590, w3629, w3634, w3589, w3622, w3634, w3585, w3627, w3634, w3583, w3618, w3634, w3580, w3619, w3634, w3577, w3633, w3634, w3574, w3637) -> (w3596:string)
                n2600 = Concatenate Strings(w3566, "," ("string"), w3554, w3556, w3555, w3638, w3641, w3555, w3639, w3640, w3566) -> (w3564:string)
                n2601 = local read "Tested by"() -> (w3570:string)
                n2602 = local read "String 33"() -> (w3571:string)
                n2603 = Concatenate Strings("," ("string"), "                                                                             " ("string")) -> (w3559:string)
                n2604 = Concatenate Strings(w3561, w3557, w3564, w3557, w3567, w3596, w3557, w3559, w3571, w3570) -> (→"export":string)
                n2605 = String To Path(string=w3598) -> (path=w3605:path)
                n2606 = local read "export"() -> (w3600:string)
                n2607 = call <vilib>:"Write Characters To File.vi"("append to file? (new file:F)"=FALSE, "character string"=w3600, "file path (dialog if empty)"=w3605) -> ()  [unwired: 2 in, 1 out]
              }
            }
          }
          frame Enabled {
          }
        }
        n2608 = case shown="True" "OK Button 17" {
          frame False {
          }
          frame True {
            (unwired) 0  # existing file
            w3858 = "Choose a datalog file to open"  # prompt
            n2609 = local write "OK Button 17"(FALSE ("OK Button 17")) -> ()
            n2610 = local read "String"() -> (w3853:string)
            n2611 = String To Path(string=w3853) -> (path=w3854:path)
            n2612 = File Dialog(6:"*.duf" ("pattern"), 7:w3858, 11:w3854) -> (0:w3845:errorcluster, 3:w3864:path)  [unwired: 4 in, 2 out]
            n2613 = Unbundle(w3845) -> ()  [unwired: 3 out]
            n2614 = Open/Create/Replace File "Open File"(file path (use dialog)=w3864) -> (refnum out=w3856:refnum<file>)  [unwired: 5 in, 2 out]
            n2615 = Strip Path(path=w3864) -> (name=w3862:string)  [unwired: 1 out]
            n2616 = Path To String(path=w3864) -> (string=w3847:string)
            n2617 = while {
              tunnel: w3856 -> [w3868]
              i -> [w3865]
              stop <- w3866 continue-if-true
              (unwired) TRUE ("line mode (F)")
              n2618 = Read from Text File "Read File"(file (use dialog)=w3868) -> (text=w3867:string)  [unwired: 3 in, 3 out]
              n2619 = local write "Numeric 16"(w3865) -> ()
              n2620 = String Length(string=w3867) -> (length=w3870:i32)
              n2621 = Greater?(x=w3870, y=1) -> (0:w3866:bool)
            }
            n2622 = local write "String 29"(w3847) -> ()
            n2623 = Search and Replace String(input string=w3847, search string=".duf", replace string=".dgf" ("replace string (\"\")")) -> (result string=→"String Indicator 4":string)  [unwired: 5 in, 3 out]
            n2624 = Match Pattern(string=w3862, regular expression=".dwm") -> (before substring=w3846:string)  [unwired: 1 in, 3 out]
            "String Indicator" <- w3846
            n2625 = Match Pattern(string=w3847, regular expression=".dwm" ("substring (\"\")")) -> (before substring=w3848:string)  [unwired: 1 in, 3 out]
            "String Indicator 3" <- w3848
            n2626 = local write "TITTLE 2"(w3846) -> ()
            n2627 = String To Path(string=w3848) -> (path=w3855:path)
            "path" <- w3855
            n2628 = call <vilib>:"Read Characters From File.vi"("file path (dialog if empty)"=w3855, "start of read offset (chars.:0)"=60 ("start of read offset (chars.: 0)")) -> ("character string"=→"String Indicator 2":string)  [unwired: 4 in, 3 out]
          }
        }
        n2629 = case shown="True" "OK Button 16" {
          frame False {
          }
          frame True {
            n2630 = stacked-sequence {
              frame #0 {
                n2631 = local read "Numeric 16"() -> (w3872:i32)
                n2632 = local write "Numeric 10"(w3872) -> ()
              }
              frame #1 {
                n2633 = local read "S.NO"() -> (→"s.NO":string)
                n2634 = local read "String 29"() -> (w3876:string)
                n2635 = String To Path(string=w3876) -> (path=w3875:path)
                n2636 = Open/Create/Replace File "Open File"(file path (use dialog)=w3875) -> (refnum out=w3877:refnum<file>)  [unwired: 5 in, 2 out]
                n2637 = for {
                  N: 16 -> [_]
                  tunnel: w3877 -> [w3884]
                  i -> [w3880]
                  (unwired) TRUE ("line mode (F)")
                  n2638 = Read from Text File "Read File"(file (use dialog)=w3884) -> (text=w3878:string)  [unwired: 3 in, 3 out]
                  n2639 = Match Pattern(string=w3878, regular expression="(") -> (after substring=w3883:string)  [unwired: 1 in, 3 out]
                  n2640 = Match Pattern(string=w3883, regular expression=")") -> (before substring=w3879:string)  [unwired: 1 in, 3 out]
                  n2641 = case shown="1" w3880 {
                    tunnel: w3879 -> [w3885 w3886 _ _ w3887 w3888 w3889 w3891 w3893 w3895 w3897 w3899 w3901 w3903 _]
                    tunnel: w3878 -> [_ _ _ _ _ _ _ _ _ _ _ _ _ _ _]
                    frame 0 {
                      "TITTLE" <- w3885
                    }
                    frame 1 {
                      "Sample ID" <- w3886
                    }
                    frame 2 {
                    }
                    frame 3 {
                    }
                    frame 4 {
                      "Test Date" <- w3887
                    }
                    frame 5 {
                      "Tested by" <- w3888
                    }
                    frame 6 {
                      n2642 = Fract/Exp String To Number(string=w3889) -> (number=→"Humidity before test 2":dbl)  [unwired: 3 in, 1 out]
                    }
                    frame 7 {
                      n2643 = Fract/Exp String To Number(string=w3891) -> (number=→"Temperature before test 2":dbl)  [unwired: 3 in, 1 out]
                    }
                    frame 8 {
                      n2644 = Fract/Exp String To Number(string=w3893) -> (number=→"Humidity after test 2":dbl)  [unwired: 3 in, 1 out]
                    }
                    frame 9 {
                      n2645 = Fract/Exp String To Number(string=w3895) -> (number=→"Temperature after test 2":dbl)  [unwired: 3 in, 1 out]
                    }
                    frame 10 {
                      n2646 = Fract/Exp String To Number(string=w3897) -> (number=→"MWSD 2":dbl)  [unwired: 3 in, 1 out]
                    }
                    frame 11 {
                      n2647 = Fract/Exp String To Number(string=w3899) -> (number=→"AVP 2":dbl)  [unwired: 3 in, 1 out]
                    }
                    frame 12 {
                      n2648 = Fract/Exp String To Number(string=w3901) -> (number=→"HCF 2":dbl)  [unwired: 3 in, 1 out]
                    }
                    frame 13 {
                      n2649 = Fract/Exp String To Number(string=w3903) -> (number=→"WS1.4 2":dbl)  [unwired: 3 in, 1 out]
                    }
                    frame 14, Default {
                    }
                  }
                }
              }
              frame #2 {
              }
            }
            n2650 = local write "OK Button 16"(FALSE ("OK Button 13")) -> ()
          }
        }
        n2651 = call <vilib>:"Query Available Printers.vi"() -> ("system configured printers"=w3547:string[])  [unwired: 9 in, 2 out]
        "System Configured Printers 2" <- w3547
        n2652 = local read "OK Button 16"() -> (w3544:bool)
        n2653 = Index Array(array=w3547, index="Select Printer 3") -> (element=w3549:string)
        "Selected Printer" <- w3549
        n2654 = case shown="True" w3544 {
          frame False {
          }
          frame True {
            n2655 = flat-sequence {
              frame #0 {
              }
              frame #1 {
                n2656 = Wait (ms)(milliseconds to wait=u32 100) -> ()  [unwired: 1 out]
              }
              frame #2 {
                n2657 = local write "OK Button 16"(FALSE ("Print 3")) -> ()
              }
            }
          }
        }
        n2658 = case shown="True" "Print" {
          tunnel: w3549 -> [_ w3841]
          frame False {
          }
          frame True {
            (unwired) i16 6 ("width (-)")
            (unwired) "TESTED BY : "
            (unwired) "TESTED DATE :"
            (unwired) "SAMPLE ID : "
            (unwired) "SAMPLE DESIGN : "
            w3799 = "\r"
            w3816 = "\r"
            # "add image"
            n2659 = local read "Sample ID"() -> (w3789:string)
            n2660 = local read "Tested by"() -> (w3792:string)
            n2661 = local read "String 34"() -> (w3779:string)
            n2662 = local read "String 45"() -> (w3759:string)
            n2663 = local read "String 35"() -> (w3774:string)
            n2664 = local read "String 37"() -> (w3772:string)
            n2665 = local read "String 32"() -> (w3794:string)
            n2666 = local read "String 36"() -> (w3769:string)
            n2667 = local read "String 31"() -> (w3793:string)
            n2668 = local read "Test Date"() -> (w3790:string)
            n2669 = local read "String 33"() -> (w3795:string)
            n2670 = local read "String 38"() -> (w3765:string)
            n2671 = local read "String 39"() -> (w3762:string)
            n2672 = local write "Print"(FALSE ("Print FF")) -> ()
            n2673 = local read "S 39"() -> (w3777:string)
            n2674 = local read "S 38"() -> (w3784:string)
            n2675 = local read "Temperature before test 2"() -> (w3815:dbl)
            n2676 = local read "Temperature after test 2"() -> (w3805:dbl)
            n2677 = local read "Humidity before test 2"() -> (w3830:dbl)
            n2678 = local read "Humidity after test 2"() -> (w3814:dbl)
            n2679 = local read "MWSD 2"() -> (w3819:dbl)
            n2680 = local read "WS1.4 2"() -> (w3797:dbl)
            n2681 = Concatenate Strings("2)" ("string"), w3779) -> (w3780:string)
            n2682 = Concatenate Strings("3)" ("string"), w3777) -> (w3778:string)
            n2683 = Concatenate Strings("1)" ("string"), w3784) -> (w3783:string)
            n2684 = Concatenate Strings("4)" ("string"), w3774) -> (w3775:string)
            n2685 = Concatenate Strings("5)" ("string"), w3772) -> (w3771:string)
            n2686 = Concatenate Strings("6)" ("string"), w3769) -> (w3768:string)
            n2687 = Concatenate Strings("7)" ("string"), w3765) -> (w3766:string)
            n2688 = Concatenate Strings("8)" ("string"), w3762) -> (w3763:string)
            n2689 = local read "HCF 2"() -> (w3801:dbl)
            n2690 = local read "AVP 2"() -> (w3818:dbl)
            n2691 = local read "s.NO"() -> (w3760:string)
            n2692 = call <vilib>:"New Report.vi"("report type"=enum16{"Standard Report", "HTML"}."Standard Report") -> ("report out"=w3839:refnum<class "NI_report.lvclass">, "error out"=w3838:errorcluster)  [unwired: 13 in]
            n2693 = local read "TITTLE"() -> (w3791:string)
            n2694 = Concatenate Strings(w3816, w3759, w3760, w3816, w3794, w3789, w3816, w3793, w3790, w3816, w3795, w3792, w3816) -> (w3809:string)
            "test by" <- w3809
            n2695 = Number To Fractional String(number=w3815, width (-)=i16 6, precision (6)=i16 2) -> (F-format string=w3804:string)  [unwired: 1 in]
            n2696 = Number To Fractional String(number=w3814, width (-)=i16 6, precision (6)=i16 2) -> (F-format string=w3817:string)  [unwired: 1 in]
